vi "RP compress sweep INT.vi"(6 "First call?":bool, 8 "Error In":errorcluster, 9 "F":i32[](array[numeric]), 10 "Y":i32[](array[numeric]), 11 "X":i32[](array[numeric])) -> (0 "Error Out":errorcluster, 1 "F out":dbl[](array[numeric]) format="%#_6p", 2 "Y out":dbl[](array[numeric]), 3 "X out":dbl[](array[numeric]))   [LabVIEW 2015]
panel:
  in  "Scale":dbl=1e-05
  out "Numeric Control":i32
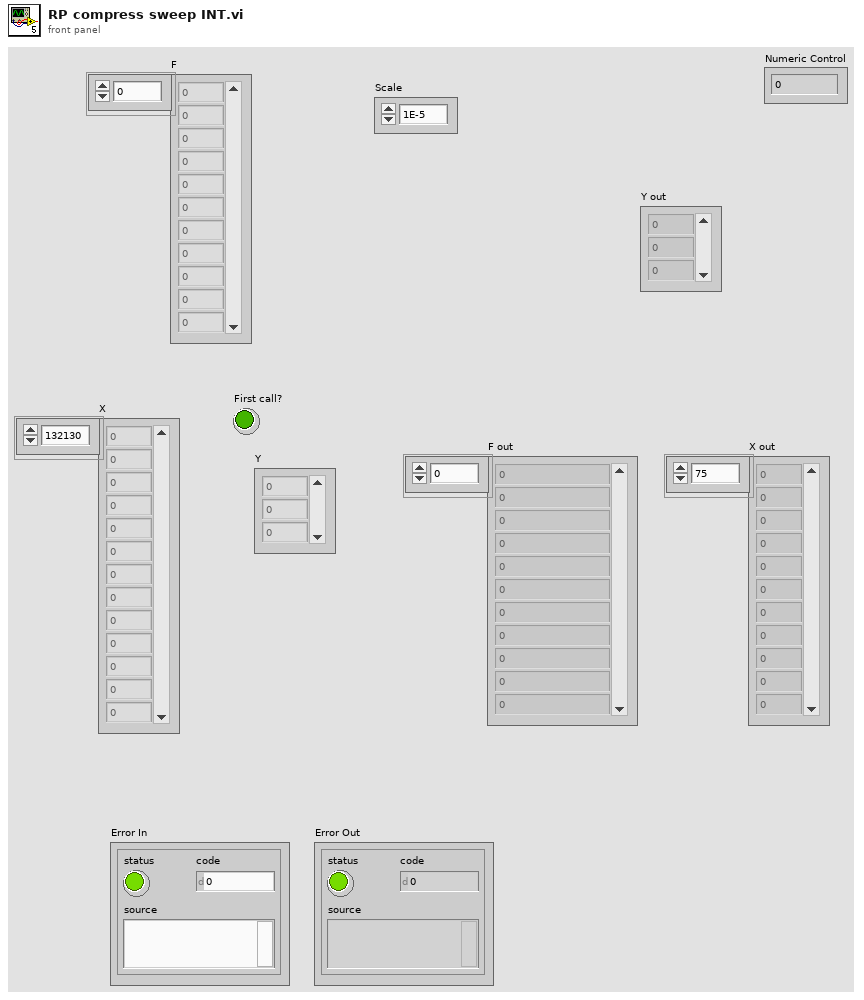
[diagram p1: front panel]
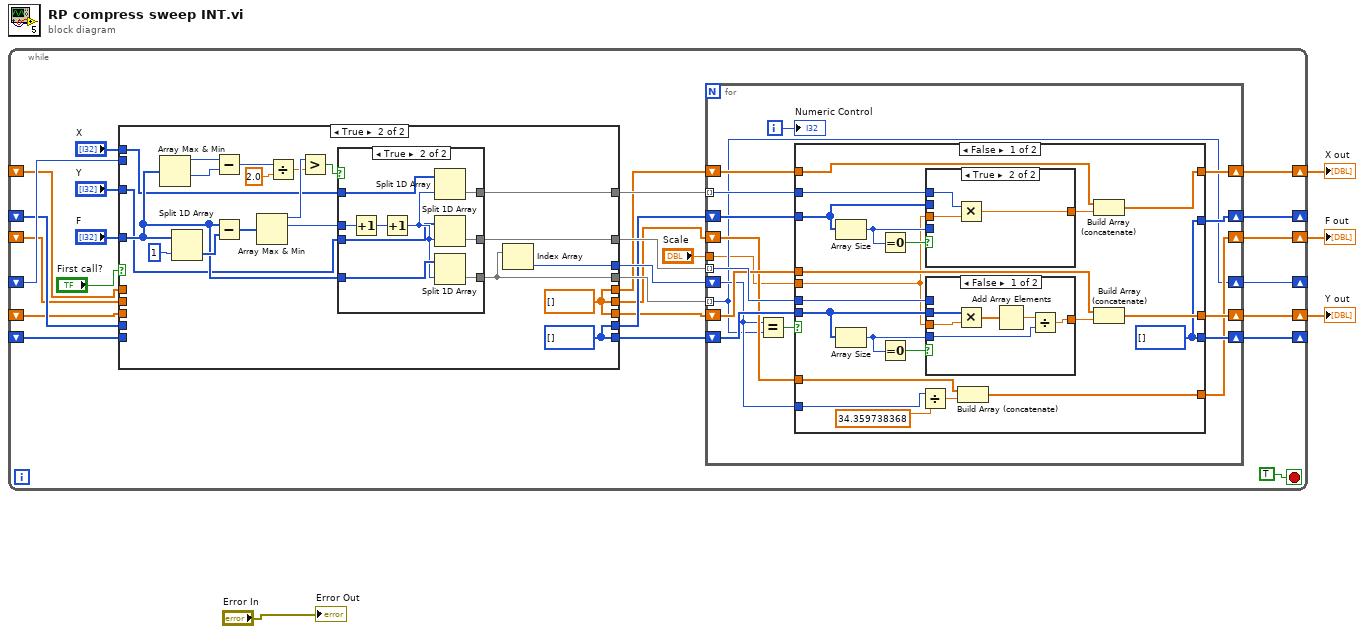
[diagram p0: block diagram]
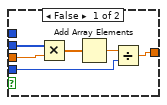
[diagram p4: hidden frame]
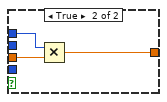
[diagram p5: hidden frame]
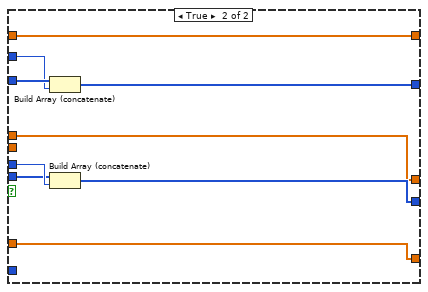
[diagram p6: hidden frame]
diagram:
  n1 = while {
    shift-right: [w17] -> _
    shift-left: _ -> [w18]
    shift-right: [w21] -> _
    shift-left: _ -> [w22]
    shift-right: [w15] -> _
    shift-left: _ -> [w16]
    shift-right: [w11] -> w4
    shift-left: _ -> [w10]
    shift-right: [w8] -> w3
    shift-left: _ -> [w9]
    shift-right: [w7] -> w2
    shift-left: _ -> [w6]
    stop <- TRUE stop-if-true
    n2 = case shown="True" "First call?" {
      tunnel: [w40 w49] -> w31
      tunnel: [w39 w48] -> w30
      tunnel: [w38 w44] -> w29
      tunnel: "F" -> [w38 w47]
      tunnel: "X" -> [w40 w46]
      tunnel: "Y" -> [w39 w45]
      tunnel: [w37 w43] -> w23
      tunnel: w22 -> [w37 _]
      tunnel: [w36 w42] -> w20
      tunnel: [w35 w42] -> w19
      tunnel: w18 -> [w36 _]
      tunnel: w16 -> [w35 _]
      tunnel: [w34 w41] -> w14
      tunnel: [w33 w41] -> w13
      tunnel: [w32 w41] -> w12
      tunnel: w10 -> [w34 _]
      tunnel: w9 -> [w33 _]
      tunnel: w6 -> [w32 _]
      frame False {
      }
      frame True {
        w41 = dbl[] [] ("Y")
        w42 = i32[] [] ("Y")
        n3 = Array Max & Min(array=w47) -> (max value=w57:i32, min value=w56:i32)  [unwired: 2 out]
        n4 = Split 1D Array(array=w47, index=1) -> (second subarray=w59:i32[])  [unwired: 1 out]
        n5 = Subtract(x=w57, y=w56) -> (x-y=w55:i32)
        n6 = Subtract(x=w47, y=w59) -> (x-y=w58:i32[])
        n7 = Array Max & Min(array=w58) -> (max value=w53:i32, max index (indices)=w50:i32)  [unwired: 2 out]
        n8 = Divide(x=w55, y=2.0) -> (x/y=w52:dbl)
        n9 = Greater?(x=w53, y=w52) -> (0:w51:bool)
        n10 = case shown="True" w51 {
          tunnel: w50 -> [_ w72]
          tunnel: w47 -> [w61 w70]
          tunnel: [w61 w69] -> w44
          tunnel: w46 -> [w62 w68]
          tunnel: [w62 w66] -> w49
          tunnel: w45 -> [w63 w65]
          tunnel: [w63 w64] -> w48
          frame False {
          }
          frame True {
            n11 = Increment(x=w72) -> (x+1=w71:i32)
            n12 = Increment(x=w71) -> (x+1=w67:i32)
            n13 = Split 1D Array(array=w68, index=w67) -> (second subarray=w66:i32[])  [unwired: 1 out]
            n14 = Split 1D Array(array=w65, index=w67) -> (second subarray=w64:i32[])  [unwired: 1 out]
            n15 = Split 1D Array(array=w70, index=w67) -> (second subarray=w69:i32[])  [unwired: 1 out]
          }
        }
        n16 = Index Array(array=w44) -> (element=w43:i32)  [unwired: 1 in]
      }
    }
    n17 = for {
      tunnel: w29 -> [w75] mode=indexing
      shift-right: [w75] -> w21
      shift-left: w23 -> [w77]
      shift-right: [w84] -> w15
      shift-left: w19 -> [w86]
      shift-right: [w85] -> w17
      shift-left: w20 -> [w89]
      tunnel: w31 -> [w88] mode=indexing
      tunnel: w30 -> [w87] mode=indexing
      shift-right: [w81] -> w11
      shift-left: w14 -> [w82]
      shift-right: [w79] -> w8
      shift-left: w13 -> [w80]
      shift-right: [w76] -> w7
      shift-left: w12 -> [w78]
      tunnel: "Scale" -> [w73]
      i -> [w74]
      n18 = Equal?(x=w77, y=w75) -> (x = y?=w83:bool)
      n19 = case shown="False" w83 {
        tunnel: w89 -> [w98 w137]
        tunnel: w88 -> [w92 w136]
        tunnel: w87 -> [w100 w135]
        tunnel: w86 -> [w110 w134]
        tunnel: [w95 w133] -> w85
        tunnel: [w95 w132] -> w84
        tunnel: w82 -> [w109 w131]
        tunnel: [w108 w131] -> w81
        tunnel: w80 -> [w107 w130]
        tunnel: [w105 w130] -> w79
        tunnel: w78 -> [w104 w129]
        tunnel: w77 -> [w90 _]
        tunnel: [w103 w129] -> w76
        tunnel: w73 -> [w94 _]
        frame False {
          w95 = i32[] [] ("Y")
          n20 = Array Size(array=w98) -> (size(s)=w96:i32)
          n21 = Array Size(array=w110) -> (size(s)=w102:i32)
          n22 = Equal To 0?(x=w96) -> (x = 0?=w99:bool)
          n23 = Equal To 0?(x=w102) -> (x = 0?=w101:bool)
          n24 = Divide(x=w90, y=34.359738368 ("x*y")) -> (x/y=w93:dbl)
          n25 = case shown="True" w99 {
            tunnel: w98 -> [w112 _]
            tunnel: [w115 w117] -> w97
            tunnel: w96 -> [w114 _]
            tunnel: w94 -> [w111 w119]
            tunnel: w92 -> [_ w118]
            frame False {
              n26 = Multiply(x=w112, y=w111) -> (x*y=w113:dbl[])
              n27 = Add Array Elements(numeric array=w113) -> (sum=w116:dbl)
              n28 = Divide(x=w116, y=w114) -> (x/y=w115:dbl)
            }
            frame True {
              n29 = Multiply(x=w118, y=w119) -> (x*y=w117:dbl)
            }
          }
          n30 = case shown="False" w101 {
            tunnel: w110 -> [w121 _]
            tunnel: [w124 w126] -> w106
            tunnel: w102 -> [w123 _]
            tunnel: w100 -> [_ w127]
            tunnel: w94 -> [w120 w128]
            frame False {
              n31 = Multiply(x=w121, y=w120) -> (x*y=w122:dbl[])
              n32 = Add Array Elements(numeric array=w122) -> (sum=w125:dbl)
              n33 = Divide(x=w125, y=w123) -> (x/y=w124:dbl)
            }
            frame True {
              n34 = Multiply(x=w127, y=w128) -> (x*y=w126:dbl)
            }
          }
          n35 = Build Array (concatenate)(w104, w93) -> (w103:dbl[])
          n36 = Build Array (concatenate)(w109, w97) -> (w108:dbl[])
          n37 = Build Array (concatenate)(w107, w106) -> (w105:dbl[])
        }
        frame True {
          n38 = Build Array (concatenate)(w137, w136) -> (w133:i32[])
          n39 = Build Array (concatenate)(w134, w135) -> (w132:i32[])
        }
      }
      "Numeric Control" <- w74
    }
  }
  "X out" <- w4
  "Y out" <- w3
  "F out" <- w2
  "Error Out" <- "Error In"
